vi "RT Main.vi"() -> (0 "error out":errorcluster)   [LabVIEW 2013]
uses:
  <vilib>/NI/Web Messaging  Palette/SubVIs/Web Messaging API.lvlib
panel:
  in  "Services Token":string="8436ac88b8807f3764b4fc96bde6d0c2174c970e"
  # "This app demonstrates how to use the myRIO Web App messaging and monitoring web site\n-Get started by visiting https://myrio.niwsc.com and creating an account\n-On the myRIO Web App click 'My account' and then click 'Services token'\n-On the Services token tab click 'Generate new token'\n-Copy your new services token and paste it in this VI's Services Token control\n-Run the VI and see that the messages and errors show up on the myRIO Web App"
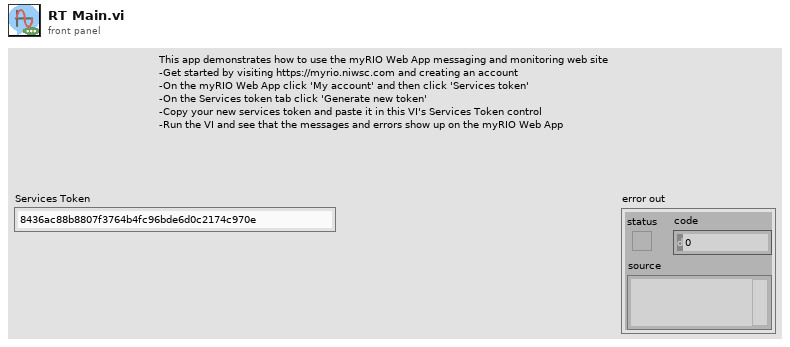
[diagram p1: front panel]
types:
  T1 = typedef "Web Messaging API.lvlib/Web Messaging Handle.ctl" = cluster{"Services token":string}
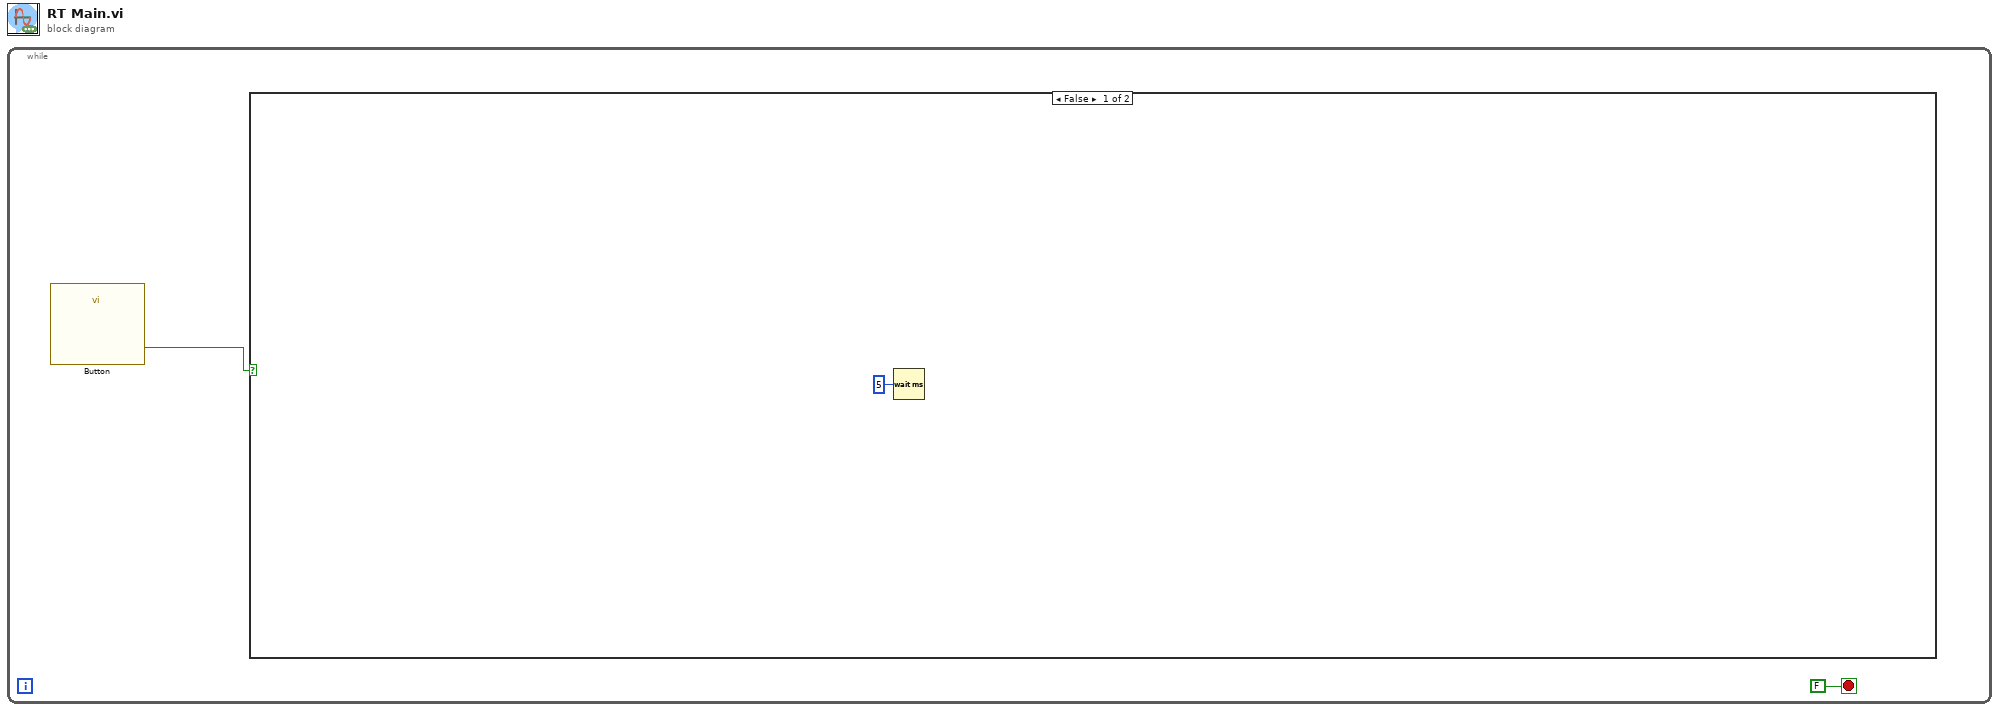
[diagram p0: block diagram]
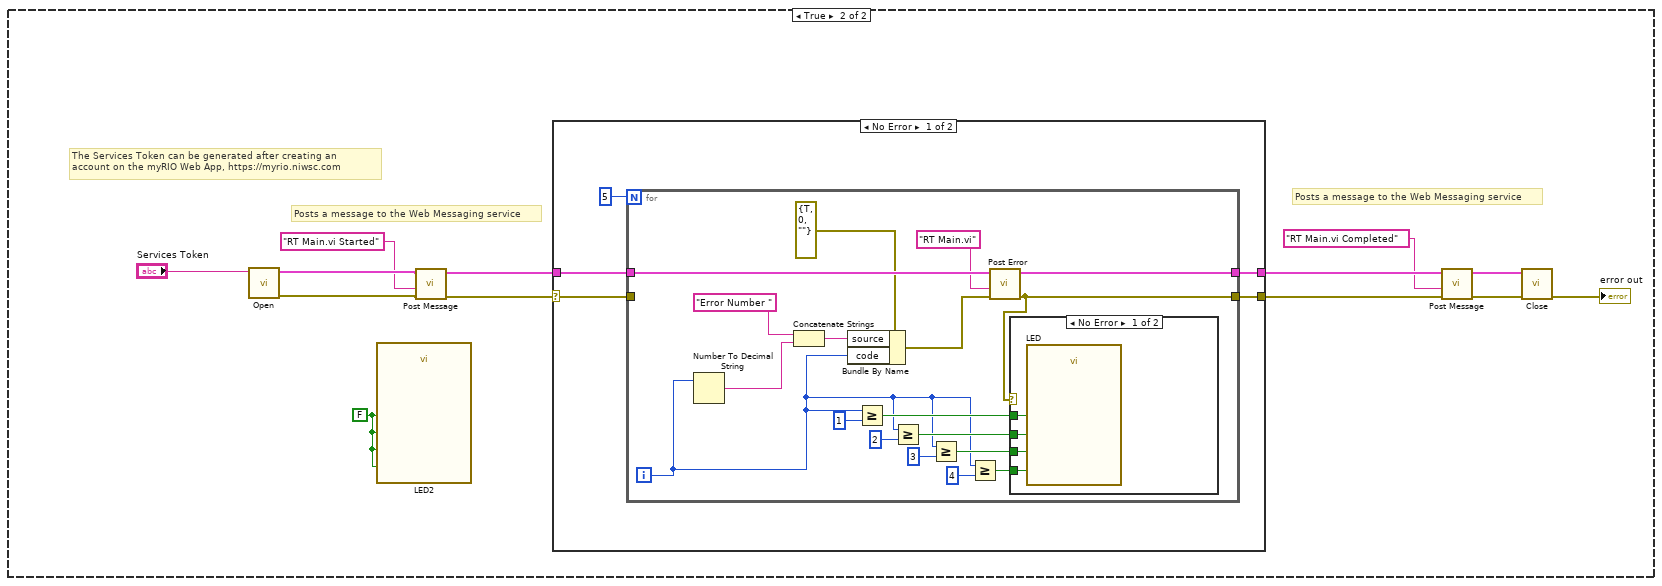
[diagram p2: hidden frame]
diagram:
  n1 = while {
    stop <- FALSE stop-if-true
    n2 = call "Button"() -> ("Value"=w1:bool)  [unwired: 26 in, 1 out]
    n3 = case shown="False" w1 {
      frame False {
        n4 = Wait (ms)(milliseconds to wait=u32 5) -> ()  [unwired: 1 out]
      }
      frame True {
        w5 = FALSE ("Error 1")
        # "Posts a message to the Web Messaging service"
        # "Posts a message to the Web Messaging service"
        # "The Services Token can be generated after creating an \naccount on the myRIO Web App, https://myrio.niwsc.com"
        n5 = call <vilib>:"Open.vi"("Services Token"="Services Token") -> ("error out"=w10:errorcluster, "Web App Handle"=w12:T1)  [unwired: 9 in]
        n6 = call "LED2"("Error 1"=w5, "Error 2"=w5, "Error 3"=w5, "Error 4"=w5) -> ()  [unwired: 23 in, 1 out]
        n7 = call <vilib>:"Post Message.vi"("error in (no error)"=w10, "message"="RT Main.vi Started", "Web App Handle In"=w12) -> ("error out"=w15:errorcluster, "Web App Handle Out"=w14:T1)  [unwired: 6 in, 1 out]
        n8 = case shown="No Error" w15 {
          selector: w15 -> [w18 w45]
          tunnel: [w17 w45] -> w16
          tunnel: w14 -> [w20 w44]
          tunnel: [w19 w44] -> w13
          frame No Error {
            n9 = for {
              N: 5 -> [_]
              tunnel: w20 -> [w39]
              tunnel: [w38] -> w19
              tunnel: w18 -> [_]
              tunnel: [w22] -> w17
              i -> [w23]
              n10 = Number To Decimal String(number=w23) -> (decimal integer string=w35:string)  [unwired: 1 in]
              n11 = Concatenate Strings("Error Number " ("string"), w35) -> (w34:string)
              n12 = Bundle By Name(cluster=errorcluster {"status"=TRUE, "code"=0, "source"=""} ("error IO"), "source"=w34, "code"=w23) -> (w33:errorcluster)
              n13 = Greater Or Equal?(x=w23, y=1) -> (x >= y?=w30:bool)
              n14 = Greater Or Equal?(x=w23, y=2) -> (x >= y?=w26:bool)
              n15 = Greater Or Equal?(x=w23, y=3) -> (x >= y?=w25:bool)
              n16 = Greater Or Equal?(x=w23, y=4) -> (x >= y?=w24:bool)
              n17 = call <vilib>:"Post Error.vi"("Web App Handle In"=w39, "message"="RT Main.vi", "error in"=w33) -> ("Web App Handle Out"=w38:T1, "error out"=w22:errorcluster)  [unwired: 5 in, 1 out]
              n18 = case shown="No Error" w22 {
                tunnel: w30 -> [w43 _]
                tunnel: w26 -> [w42 _]
                tunnel: w25 -> [w41 _]
                tunnel: w24 -> [w40 _]
                frame No Error {
                  n19 = call "LED"("Error 1"=w43, "Error 2"=w42, "Error 3"=w41, "Error 4"=w40) -> ()  [unwired: 23 in, 1 out]
                }
                frame Error {
                }
              }
            }
          }
          frame Error {
          }
        }
        n20 = call <vilib>:"Post Message.vi"("error in (no error)"=w16, "message"="RT Main.vi Completed", "Web App Handle In"=w13) -> ("error out"=w7:errorcluster, "Web App Handle Out"=w6:T1)  [unwired: 6 in, 1 out]
        n21 = call <vilib>:"Close.vi"("error in"=w7, "Web App Handle"=w6) -> ("error out"=→"error out":errorcluster)  [unwired: 9 in]
      }
    }
  }
